vi "FTS Get Instrument Property hwSort.vi"() -> ()   [LabVIEW 2010, in "FTSLib.lvlib"]
uses:
  FTSLib.lvlib
  FTSLib.dll
panel:
  in  "channel":u16
  out "error out":errorcluster
  in  "error in (no error)":errorcluster
  in  "autoGain":bool
  in  "specIndex":u16
  out "function return":i32
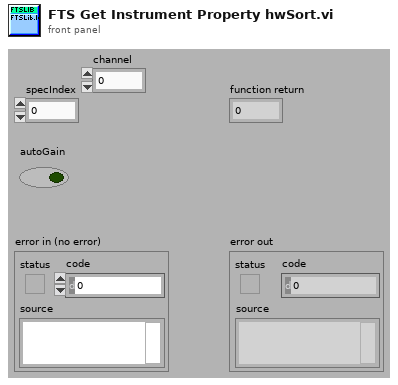
[diagram p1: front panel]
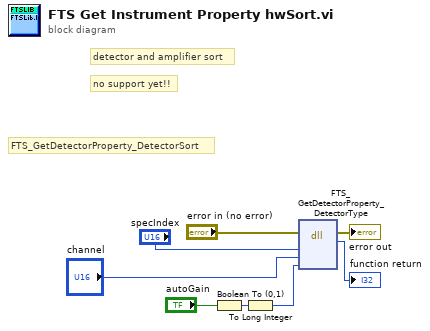
[diagram p0: block diagram]
diagram:
  # "FTS_GetDetectorProperty_DetectorSort"
  # "detector and amplifier sort"
  # "no support yet!!"
  n1 = Boolean To (0,1)(Boolean="autoGain") -> (0, 1=w5:i16)
  n2 = To Long Integer(number=w5) -> (32bit integer=w2:i32)
  n3 = dll-call lib="FTSLib.*" fn="FTS_GetDetectorProperty_DetectorType"(error in="error in (no error)", "specIndex"="specIndex", "channel"="channel", "autoGain"=w2) -> (error out=→"error out":errorcluster, "return type"=→"function return":i32)  [unwired: 5 in, 1 out]
